vi "Animate_Backup.vi"(4 "heading":dbl, 5 "xy_position":dbl[](array[numeric])=[0.0, 0.0], 6 "error in (no error)":errorcluster, 7 "Steer Angle":dbl, 8 "Car Speed":dbl, 9 "task in":refnum<class "Visualization.lvclass">) -> (2 "error out":errorcluster, 3 "task out":refnum<class "Visualization.lvclass">)   [LabVIEW 2011]
uses:
  <vilib>/Quanser/Rapid Control Prototyping Toolkit/visualization/Visualization.lvclass
  <vilib>/Quanser/Rapid Control Prototyping Toolkit/sources/CL Sample Time.vi
  <vilib>/Simulation/Implementation/Shared/SIMSCR Execution Mode.ctl
  <vilib>/Simulation/Scripting/Companion Diagram/SimConfigNode/SimParams.ctl
  <vilib>/Simulation/Scripting/Companion Diagram/SimConfigNode/_simSolvers.ctl
  <vilib>/Simulation/Param Hierarchy/Typedefs/SIMPH Param Control Actions.ctl
  <vilib>/Simulation/Utility/Implementation/NILVSim Memory.llb/NILVSim Memory (core).vi
  <vilib>/Simulation/Implementation/Shared/NILVSim_Manager.vi
  <vilib>/Simulation/Implementation/Shared/NILVSim_ParamChanged.vi
  <vilib>/Simulation/Implementation/Shared/NILVSim_FinalizeModel.vi
  <vilib>/Simulation/Implementation/Shared/SIM Unbundle Sim Info.vi
  <vilib>/Simulation/Implementation/Shared/NILVSim_GetModelError.vi
  <vilib>/Simulation/Implementation/Shared/SIM SimErrorHandler.vi
  <vilib>/Simulation/Implementation/Shared/SIM Bundle Sim Info.vi
  <vilib>/Simulation/Implementation/Shared/NILVSim_Initialize.vi
  <vilib>/Quanser/Rapid Control Prototyping Toolkit/visualization/Visualization Set Variable (1D SGL).vi
  <vilib>/Quanser/Rapid Control Prototyping Toolkit/visualization/Visualization Set Variable (2D SGL).vi
  <vilib>/imath/engines/lvmath2/RunTimeEngine/NodeEndStatement/NIMS_NodeEndStatement_Output.vi
  <instcachedir>/0/NIMS_NodeEndStatement_Output_53EC0D466D134D7ABD903AC30B43404B.lvgen/NIMS_NodeEndStatement_Output_53EC0D466D134D7ABD903AC30B43404B_005.vi
  <vilib>/imath/engines/lvmath2/RunTimeEngine/ErrorHandling/NIMS_Finalize Error.vi
  <vilib>/imath/engines/lvmath2/RunTimeEngine/VariableToken/Read/NIMS_Get Elements - RV(_) - Check.vi
  <instcachedir>/0/NIMS_Get Elements - RV(_) - Check_B511B9D8E05044FE80F9F088FE24B20C.lvgen/NIMS_Get Elements - RV(_) - Check_B511B9D8E05044FE80F9F088FE24B20C_000.vi
  <vilib>/imath/engines/lvmath2/RunTimeEngine/ErrorHandling/NIMS_Create Error From Enums.vi
  <vilib>/imath/engines/lvmath2/RunTimeEngine/NodeEndStatement/NIMS_NodeEndStatement_Get Vector.vi
  <instcachedir>/0/NIMS_NodeEndStatement_Get Vector_50E2F48DC826428EA11CD85545CBACBE.lvgen/NIMS_NodeEndStatement_Get Vector_50E2F48DC826428EA11CD85545CBACBE_001.vi
  <vilib>/imath/engines/lvmath/Functions/Error Handling/MergeErrorsWrapper.vi
  <instcachedir>/0/NIMS_NodeEndStatement_Output_53EC0D466D134D7ABD903AC30B43404B.lvgen/NIMS_NodeEndStatement_Output_53EC0D466D134D7ABD903AC30B43404B_002.vi
  <vilib>/imath/engines/lvmath2/RunTimeEngine/ArithmeticOperatorToken/NIMS_ArithmeticOperator_multmx(M,CV)-internal.vi
  <instcachedir>/0/NIMS_ArithmeticOperator_multmx(M,CV)-internal_6CB099094BC24B14AC18398D450D9232.lvgen/NIMS_ArithmeticOperator_multmx(M,CV)-internal_6CB099094BC24B14AC18398D450D9232_002.vi
  <vilib>/imathl/engines/lvmath/Functions/Error Handling/Create Error.vi
  <vilib>/imath/engines/lvmath2/RunTimeEngine/VariableToken/Read/NIMS_Get Elements - V(S).vi
  <instcachedir>/0/NIMS_Get Elements - V(S)_C99A26467DB24FA3A79619D034B25FD8.lvgen/NIMS_Get Elements - V(S)_C99A26467DB24FA3A79619D034B25FD8_000.vi
  <vilib>/imath/engines/lvmath2/RunTimeEngine/BuiltInFunctions/atan2/NIMS_atan2.vi
  <instcachedir>/0/NIMS_atan2_A91AA4A7D42247EDBE8F76DB99AF04A4.lvgen/NIMS_atan2_A91AA4A7D42247EDBE8F76DB99AF04A4_001.vi
  <vilib>/imath/engines/lvmath2/RunTimeEngine/ArithmeticOperatorToken/NIMS_ArithmeticOperator_multmx-internal.vi
  <instcachedir>/0/NIMS_ArithmeticOperator_multmx-internal_2691130F3AF84DE39DAB83523BB19DB3.lvgen/NIMS_ArithmeticOperator_multmx-internal_2691130F3AF84DE39DAB83523BB19DB3_004.vi
  <instcachedir>/0/NIMS_ArithmeticOperator_multmx-internal_2691130F3AF84DE39DAB83523BB19DB3.lvgen/NIMS_ArithmeticOperator_multmx-internal_2691130F3AF84DE39DAB83523BB19DB3_000.vi
  <vilib>/imath/engines/lvmath2/RunTimeEngine/RangeToken/NIMS_Range_R2.vi
  <vilib>/imath/engines/lvmath2/RunTimeEngine/ReplaceToken/NIMS_Replace - Check Row.vi
  <instcachedir>/0/NIMS_Replace - Check Row_3A4697C4AEF9488082381CE5531B405A.lvgen/NIMS_Replace - Check Row_3A4697C4AEF9488082381CE5531B405A_001.vi
  <vilib>/imath/engines/lvmath2/RunTimeEngine/ReplaceToken/NIMS_Replace - Check Column.vi
  <instcachedir>/0/NIMS_Replace - Check Column_7A54AC4688FE427CA8C7A22E1199AA47.lvgen/NIMS_Replace - Check Column_7A54AC4688FE427CA8C7A22E1199AA47_001.vi
  <vilib>/imath/engines/lvmath2/RunTimeEngine/VariableToken/Read/NIMS_Get Elements - CV(_) - Check.vi
  <instcachedir>/0/NIMS_Get Elements - CV(_) - Check_4CF014B95B49446692066C44E7C19A08.lvgen/NIMS_Get Elements - CV(_) - Check_4CF014B95B49446692066C44E7C19A08_005.vi
  <vilib>/imath/engines/lvmath2/RunTimeEngine/ReplaceToken/NIMS_Replace - Size Check M(_,_)=VorM.vi
  <instcachedir>/0/NIMS_Replace - Size Check M(_,_)=VorM_DBF064A3787B4BA1B9E4CE97BAD98A28.lvgen/NIMS_Replace - Size Check M(_,_)=VorM_DBF064A3787B4BA1B9E4CE97BAD98A28_029.vi
  <vilib>/imath/engines/lvmath2/RunTimeEngine/ReplaceToken/NIMS_Replace - Assignment Check M(_,_)=VorM.vi
  <instcachedir>/0/NIMS_Replace - Assignment Check M(_,_)=VorM_D7A940CD4A4243D3ACFF07414B4E3644.lvgen/NIMS_Replace - Assignment Check M(_,_)=VorM_D7A940CD4A4243D3ACFF07414B4E3644_029.vi
  <vilib>/imath/engines/lvmath2/RunTimeEngine/ArithmeticOperatorToken/NIMS_ArithmeticOperator_multmx.vi
  <instcachedir>/0/NIMS_ArithmeticOperator_multmx_7C179C1E3F6A47AEB223A71AB1A54D0B.lvgen/NIMS_ArithmeticOperator_multmx_7C179C1E3F6A47AEB223A71AB1A54D0B_004.vi
  <vilib>/imath/engines/lvmath2/RunTimeEngine/VariableToken/Read/NIMS_Get Elements - SorM(_,_) - Check - Check.vi
  <instcachedir>/0/NIMS_Get Elements - SorM(_,_) - Check - Check_DA1E252EAB634D989357E7C72E8137F5.lvgen/NIMS_Get Elements - SorM(_,_) - Check - Check_DA1E252EAB634D989357E7C72E8137F5_006.vi
  <vilib>/imath/engines/lvmath2/RunTimeEngine/ArithmeticOperatorToken/NIMS_ArithmeticOperator_plus.vi
  <instcachedir>/0/NIMS_ArithmeticOperator_plus_1E95F7DAB906458CBECCADBE8E6FD739.lvgen/NIMS_ArithmeticOperator_plus_1E95F7DAB906458CBECCADBE8E6FD739_003.vi
  <instcachedir>/0/NIMS_Replace - Size Check M(_,_)=VorM_DBF064A3787B4BA1B9E4CE97BAD98A28.lvgen/NIMS_Replace - Size Check M(_,_)=VorM_DBF064A3787B4BA1B9E4CE97BAD98A28_030.vi
  <instcachedir>/0/NIMS_Replace - Assignment Check M(_,_)=VorM_D7A940CD4A4243D3ACFF07414B4E3644.lvgen/NIMS_Replace - Assignment Check M(_,_)=VorM_D7A940CD4A4243D3ACFF07414B4E3644_030.vi
  <instcachedir>/0/NIMS_NodeEndStatement_Output_53EC0D466D134D7ABD903AC30B43404B.lvgen/NIMS_NodeEndStatement_Output_53EC0D466D134D7ABD903AC30B43404B_001.vi
  <vilib>/Simulation/Scripting/Companion Diagram/SimConfigNode/SimDog.xnode
  <vilib>/Simulation/Implementation/XNodeFramework/SimXNode/SimX.xnode
  <vilib>/Simulation/Implementation/Shared/NI_SIM_Implementation.lvlib
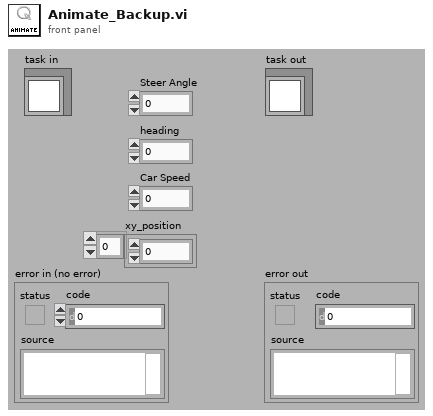
[diagram p1: front panel]
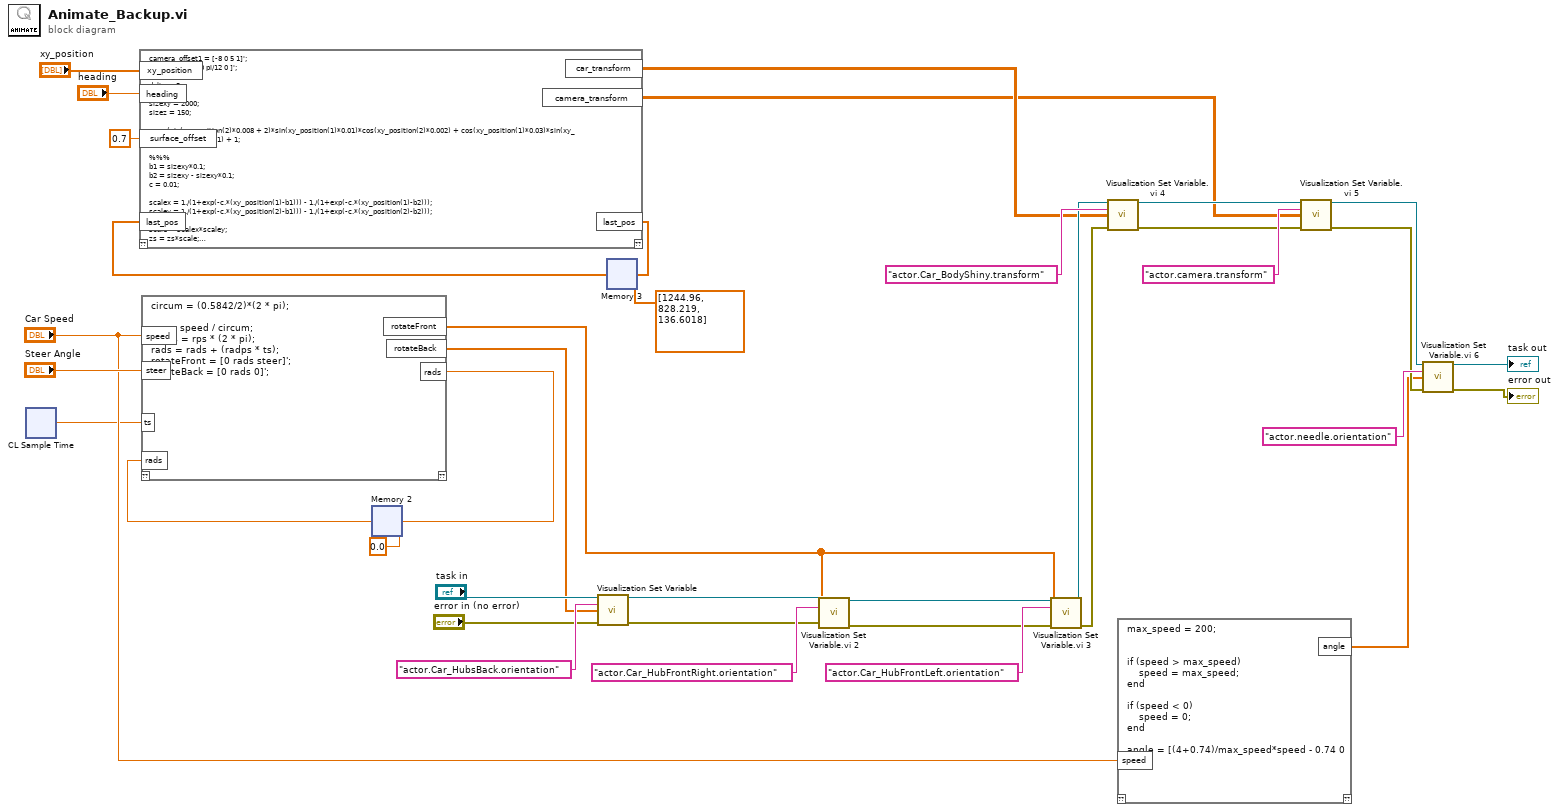
[diagram p0: block diagram]
diagram:
  n1 = xnode "CL Sample Time"() -> ("time (seconds)"=w6:dbl)
  n2 = mathscript code="max_speed = 200;\n\n\nif (speed > max_speed)\n    speed = max_speed;\nend\n\nif (speed < 0)\n    speed = 0;\nend\n\nangle = [(4+0.74)/max_speed*speed - 0.74 0 0]';"("speed"="Car Speed") -> ("angle"=w1:dbl[])  [unwired: 1 in, 1 out]
  n3 = mathscript code="camera_offset1 = [-8 0 5 1]';\nviewangle1 = [0 pi/12 0 ]';\n\ndelta = 5;\n\nsizexy = 2000;\nsizez = 150;\n\nzs = (sin(xy_position(2)*0.008 + 2)*sin(xy_position(1)*0.01)*cos(xy_position(2)*0.002) + cos(xy_position(1)*0.03)*sin(xy_position(2)*0.04)*0.1) + 1;\n\n%%%\nb1 = sizexy*0.1;\nb2 = sizexy - sizexy*0.1;\nc = 0.01;\n\nscalex = 1./(1+exp(-c.*(xy_position(1)-b1))) - 1./(1+exp(-c.*(xy_position(1)-b2)));\nscaley = 1./(1+exp(-c.*(xy_position(2)-b1))) - 1./(1+exp(-c.*(xy_position(2)-b2)));\n\nscale = scalex*scaley;\nzs = zs*scale;\n\nzs = zs*0.5*sizez;\n\nvecN = [delta 0]';\nvecE = [0 delta]';\n\nrot_z = [cos(heading) -sin(heading); sin(heading) cos(heading)];\nvecN = rot_z*vecN;\nvecE = rot_z*vecE;\n\n%%%%\nzN = (sin((vecN(2) + xy_position(2))*0.008 + 2)*sin((vecN(1) + xy_position(1))*0.01)*cos((vecN(2) + xy_position(2))*0.002) + cos((vecN(1) + xy_position(1))*0.03)*sin((vecN(2) + xy_position(2))*0.04)*0.1) + 1;\n\nscalex = 1./(1+exp(-c.*((vecN(1) + xy_position(1))-b1))) - 1./(1+exp(-c.*((vecN(1) + xy_position(1))-b2)));\nscaley = 1./(1+exp(-c.*((vecN(2) + xy_position(2))-b1))) - 1./(1+exp(-c.*((vecN(2) + xy_position(2))-b2)));\n\nscale = scalex*scaley;\nzN = zN*scale;\nzN = zN*0.5*sizez;\n\n%%%%\nzE = (sin((vecE(2) + xy_position(2))*0.008 + 2)*sin((vecE(1) + xy_position(1))*0.01)*cos((vecE(2) + xy_position(2))*0.002) + cos((vecE(1) + xy_position(1))*0.03)*sin((vecE(2) + xy_position(2))*0.04)*0.1) + 1;\n\nscalex = 1./(1+exp(-c.*((vecE(1) + xy_position(1))-b1))) - 1./(1+exp(-c.*((vecE(1) + xy_position(1))-b2)));\nscaley = 1./(1+exp(-c.*((vecE(2) + xy_position(2))-b1))) - 1./(1+exp(-c.*((vecE(2) + xy_position(2))-b2)));\n\nscale = scalex*scaley;\nzE = zE*scale;\nzE = zE*0.5*sizez;\n%%%%\n\nrx = atan2(zE-zs, delta);\nry = -atan2(zN-zs, delta);\n%%%%%\n\nz = zs;\n\nrot_x = [1 0 0 0; 0 cos(rx) -sin(rx) 0; 0 sin(rx) cos(rx) 0; 0 0 0 1];\nrot_y = [cos(ry) 0 sin(ry) 0; 0 1 0 0; -sin(ry) 0 cos(ry) 0; 0 0 0 1];\nrot_z = [cos(heading) -sin(heading) 0 0; sin(heading) cos(heading) 0 0; 0 0 1 0; 0 0 0 1];\n\noverhead_view = ([1 0 0 xy_position(1); 0 1 0 xy_position(2); 0 0 1 z+5; 0 0 0 1]*rot_z*rot_y*rot_x)*[20 0 0 0; 0 20 0 0; 0 0 20 0; 0 0 0 1];\ncar_transform = [1 0 0 xy_position(1); 0 1 0 xy_position(2); 0 0 1 z+surface_offset; 0 0 0 1]*rot_z*rot_y*rot_x;\n\nrot_x_view1 = [1 0 0 0; 0 cos(viewangle1(1)) -sin(viewangle1(1)) 0; 0 sin(viewangle1(1)) cos(viewangle1(1)) 0; 0 0 0 1];\nrot_y_view1 = [cos(viewangle1(2)) 0 sin(viewangle1(2)) 0; 0 1 0 0; -sin(viewangle1(2)) 0 cos(viewangle1(2)) 0; 0 0 0 1];\nrot_z_view1 = [cos(viewangle1(3)) -sin(viewangle1(3)) 0 0; sin(viewangle1(3)) cos(viewangle1(3)) 0 0; 0 0 1 0; 0 0 0 1];\nbackview_transform = rot_z_view1*rot_y_view1*rot_x_view1;\nbackview_transform(1:3,4) = camera_offset1(1:3);\ncamera_transform = [1 0 0 xy_position(1); 0 1 0 xy_position(2); 0 0 1 z+surface_offset; 0 0 0 1]*rot_z*backview_transform;\ncam_pos = camera_transform(1:3,4);\n\nfilter_weight = 0.05;\ncam_pos_filtered = last_pos*(1.0 - filter_weight) + filter_weight*cam_pos;\nlast_pos = cam_pos_filtered;\n\ncamera_transform(1:3,4) = cam_pos_filtered;\n\nslope = -ry;"("xy_position"="xy_position", "heading"="heading", "surface_offset"=0.7, "last_pos"=w14) -> ("last_pos"=w16:dbl[], "car_transform"=w5:dbl[][], "camera_transform"=w4:dbl[][])  [unwired: 1 in, 1 out]
  n4 = xnode ("Memory 3")("input"=w16, "initial value"=dbl[] [1244.96, 828.219, 136.6018]) -> ("output"=w14:dbl[])  [unwired: 4 in]
  n5 = mathscript code="circum = (0.5842/2)*(2 * pi);\n\nrps = speed / circum;\nradps = rps * (2 * pi);\nrads = rads + (radps * ts);\nrotateFront = [0 rads steer]';\nrotateBack = [0 rads 0]';"("speed"="Car Speed", "steer"="Steer Angle", "ts"=w6, "rads"=w25) -> ("rotateFront"=w3:dbl[], "rotateBack"=w2:dbl[], "rads"=w27:dbl)  [unwired: 1 in, 1 out]
  n6 = xnode ("Memory 2")("input"=w27, "initial value"=0.0) -> ("output"=w25:dbl)  [unwired: 4 in]
  n7 = call-poly <vilib>:"Visualization Set Variable.vi"("visualization in"="task in", "variable name"="actor.Car_HubsBack.orientation", "values"=w2, "error in (no error)"="error in (no error)") -> ("visualization out"=w31:refnum<class "Visualization.lvclass">, "error out"=w33:errorcluster)  [unwired: 10 in]
  n8 = call-poly "Visualization Set Variable.vi 2"("visualization in"=w31, "variable name"="actor.Car_HubFrontRight.orientation", "values"=w3, "error in (no error)"=w33) -> ("visualization out"=w30:refnum<class "Visualization.lvclass">, "error out"=w32:errorcluster)  [unwired: 10 in]
  n9 = call-poly "Visualization Set Variable.vi 3"("visualization in"=w30, "variable name"="actor.Car_HubFrontLeft.orientation", "values"=w3, "error in (no error)"=w32) -> ("visualization out"=w22:refnum<class "Visualization.lvclass">, "error out"=w23:errorcluster)  [unwired: 10 in]
  n10 = call-poly "Visualization Set Variable.vi 4"("visualization in"=w22, "variable name"="actor.Car_BodyShiny.transform", "values"=w5, "error in (no error)"=w23) -> ("visualization out"=w21:refnum<class "Visualization.lvclass">, "error out"=w20:errorcluster)  [unwired: 10 in]
  n11 = call-poly "Visualization Set Variable.vi 5"("visualization in"=w21, "variable name"="actor.camera.transform", "values"=w4, "error in (no error)"=w20) -> ("visualization out"=w9:refnum<class "Visualization.lvclass">, "error out"=w10:errorcluster)  [unwired: 10 in]
  n12 = call-poly "Visualization Set Variable.vi 6"("visualization in"=w9, "variable name"="actor.needle.orientation", "values"=w1, "error in (no error)"=w10) -> ("visualization out"=→"task out":refnum<class "Visualization.lvclass">, "error out"=→"error out":errorcluster)  [unwired: 10 in]
